vi "main.vi"() -> ()   [LabVIEW 2014]
uses:
  control/DEF-LabVIEW INFO.ctl
  control/DEF-State.ctl
  shared/miscellaneous.llb/miscellaneous.lvlib
panel:
  out "Symbol Found?":bool
  out "Selected Version":string
  out "Version List":string[](array[string])
  out "Symbol Path":path
  out "Symbol Version":string
  out "LabVIEW Info":T1[](array[typedef])
  in  "Cancel":bool
  in  "OK":bool
  in  "LabVIEW List":string(combo)
  in  "file path":path=path "D:/Projects/Personal/Multi-LabVIEW-Selector/Multi-LabVIEW Selector.lvproj" caption="打开文件路径"
  out "CMD line":string caption="命令行参数"
  # "主界面，所有的界面操作都产生消息，推送给Message Framework 处理。"
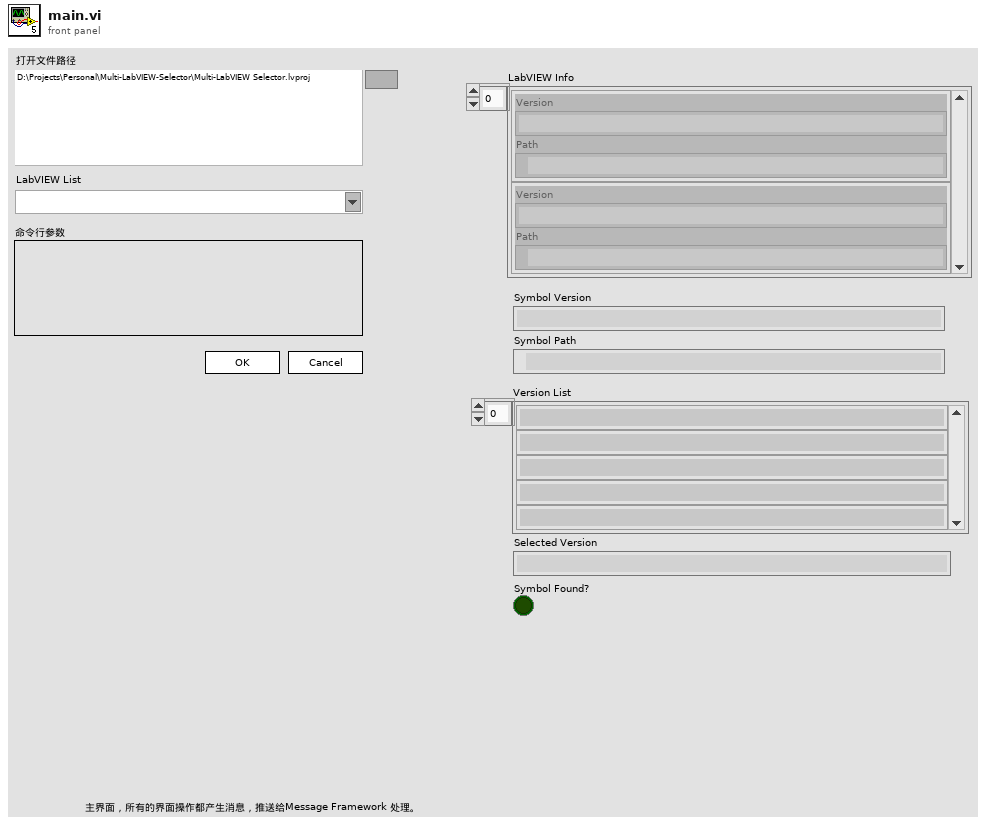
[diagram p1: front panel]
types:
  T1 = typedef "DEF-LabVIEW INFO.ctl" = cluster{"Version":string, "Path":path}
  T2 = typedef "DEF-State.ctl" = enum16{"Get Project Path", "Get Installed LabVIEW Version", "Find New Symbol", "Find Old Symbol", "Replace with New Symbol", "Check If The Symbol Version Exist", "Waiting for User Selection", "Display Information", "Open With Selected LabVIEW Version", "Exit"}
  T3 = cluster{"Project Path":path, "LabVIEW Info":T1[], "Symbol Version":string, "Symbol Path":path, "Version List":string[], "Selected Version":string, "Symbol Found?":bool, "CMD line":string}
  T4 = enum8{"Enabled", "Disabled", "Disabled and Grayed Out"}
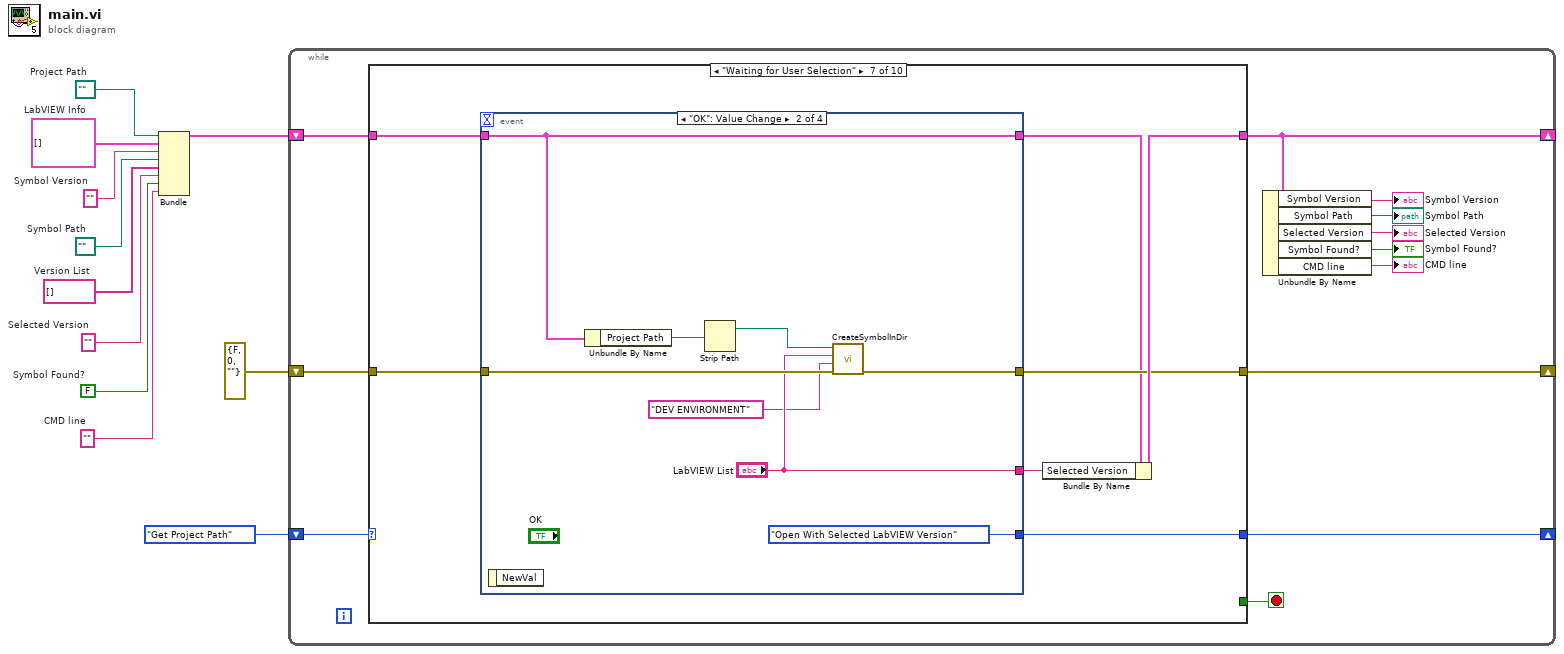
[diagram p0: block diagram]
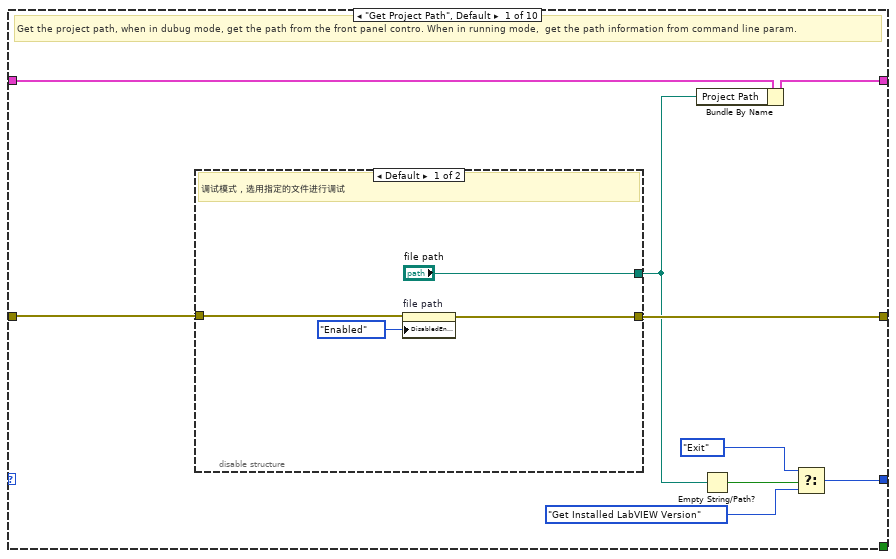
[diagram p2: hidden frame]
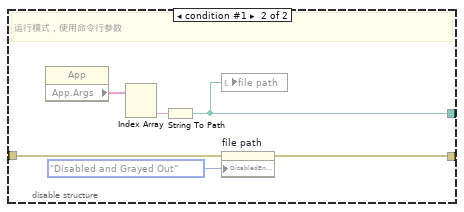
[diagram p3: hidden frame]
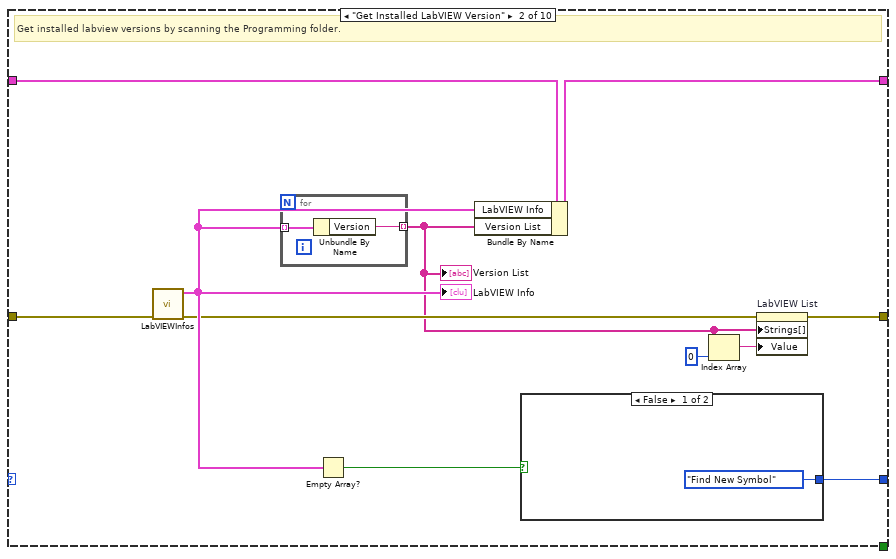
[diagram p4: hidden frame]
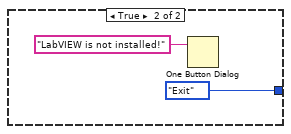
[diagram p5: hidden frame]
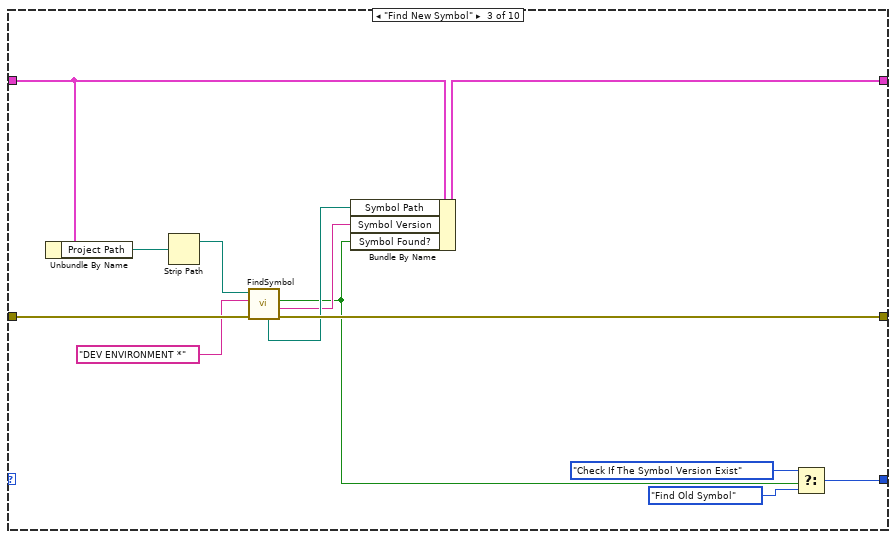
[diagram p6: hidden frame]
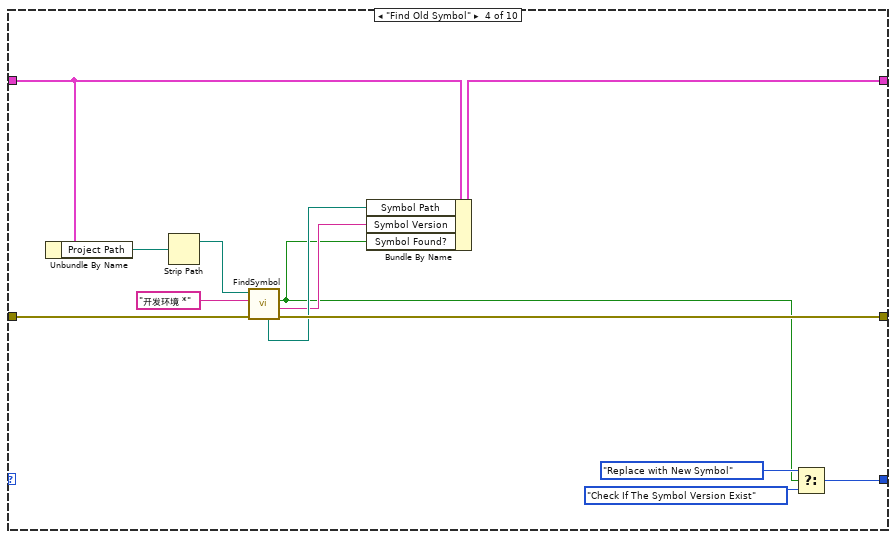
[diagram p7: hidden frame]
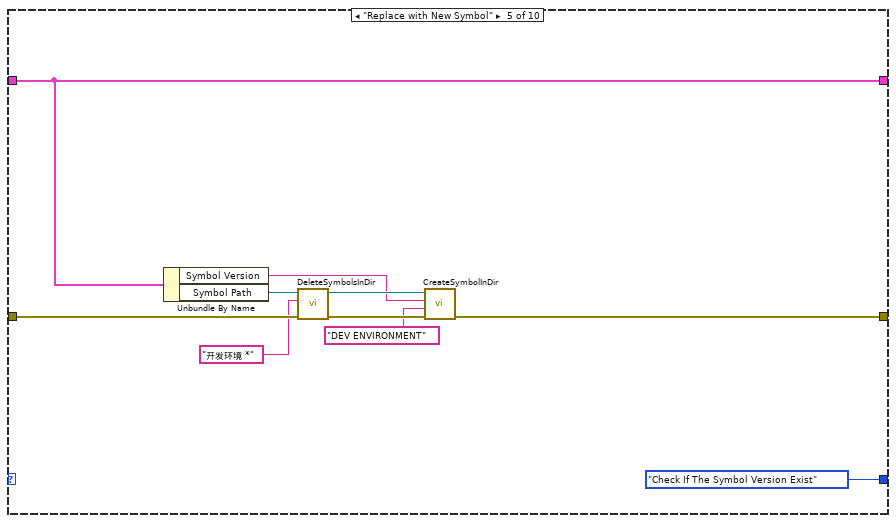
[diagram p8: hidden frame]
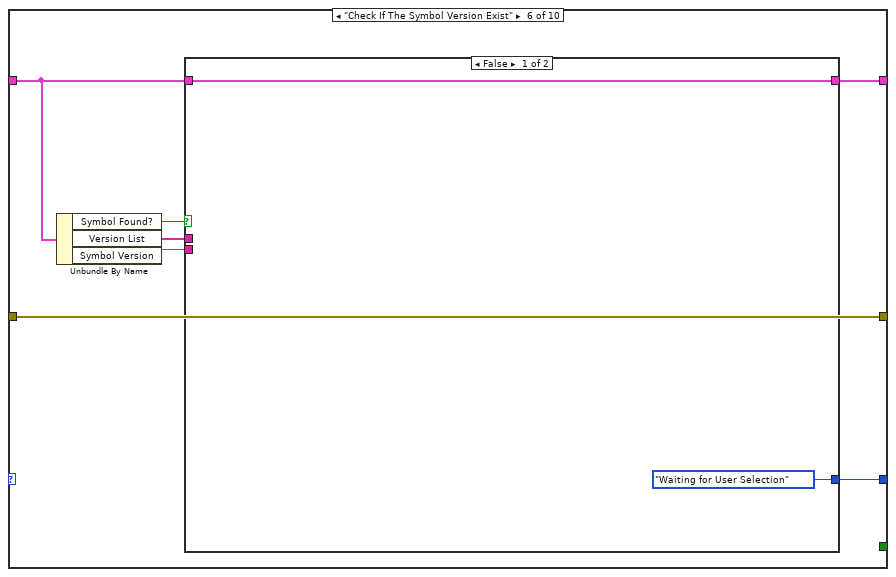
[diagram p9: hidden frame]
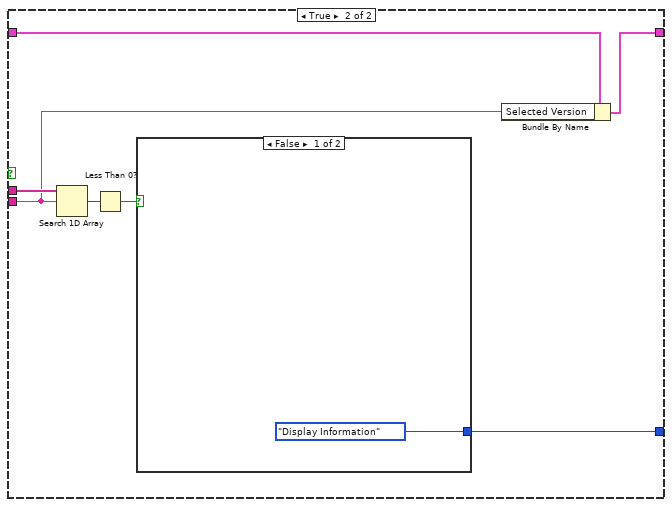
[diagram p10: hidden frame]
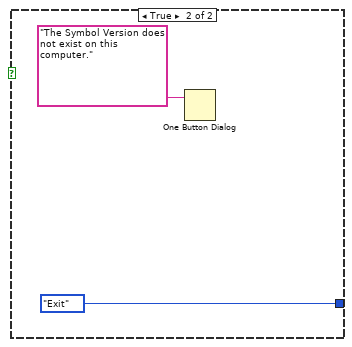
[diagram p11: hidden frame]
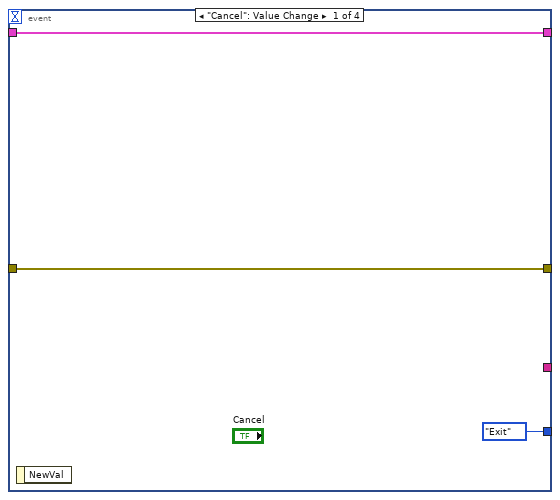
[diagram p12: hidden frame]
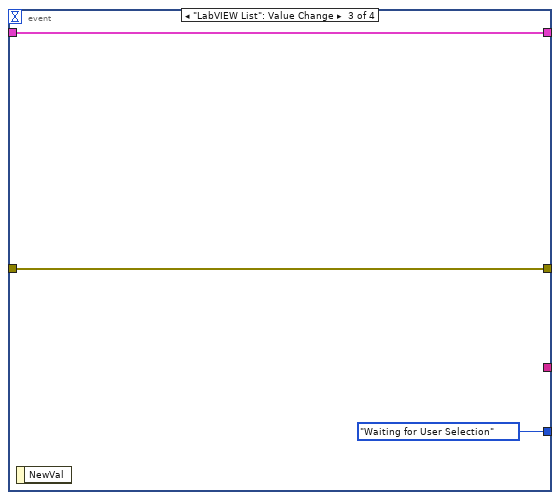
[diagram p13: hidden frame]
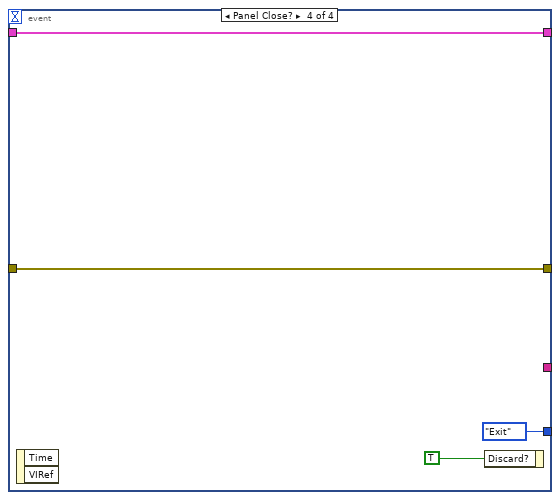
[diagram p14: hidden frame]
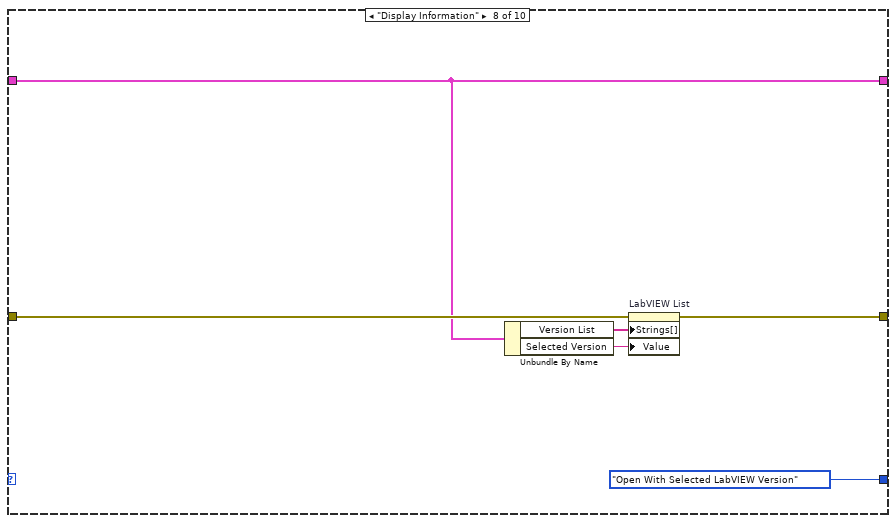
[diagram p15: hidden frame]
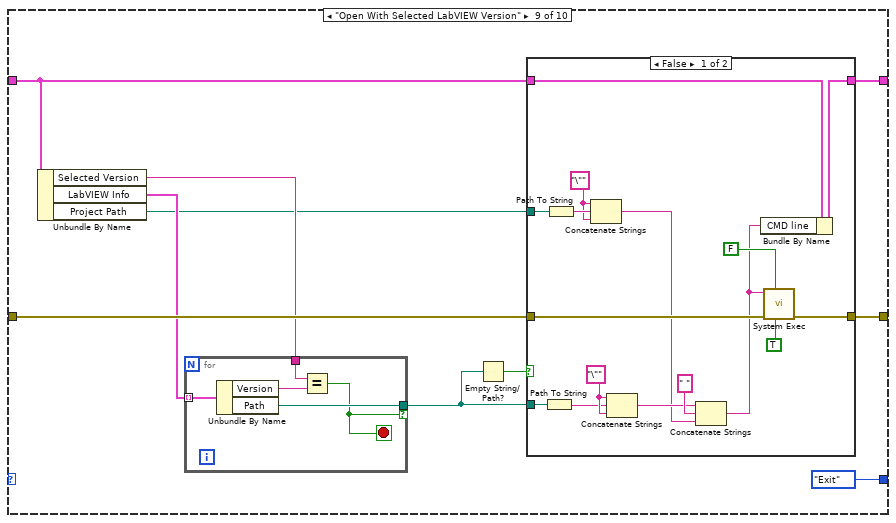
[diagram p16: hidden frame]
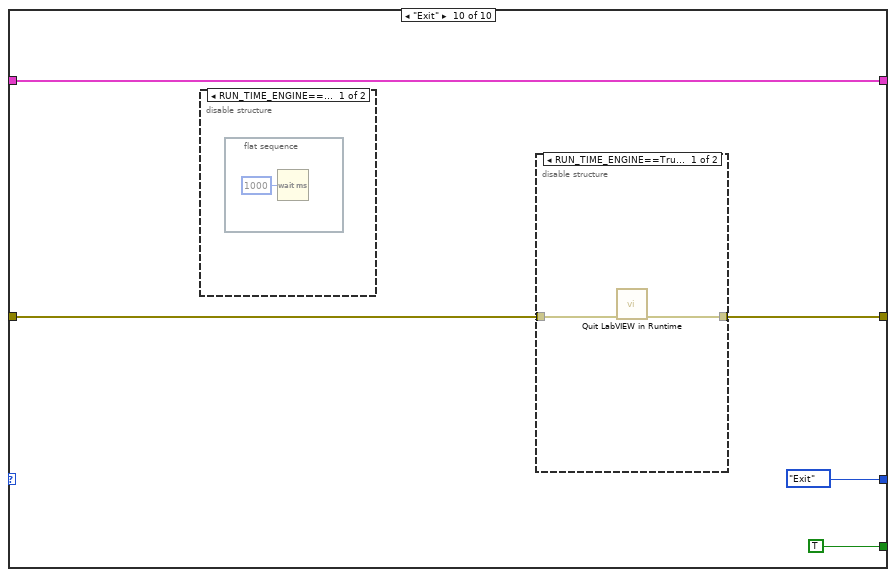
[diagram p18: hidden frame]
diagram:
  w1 = ""  # CMD line
  w2 = FALSE  # Symbol Found?
  w3 = ""  # Selected Version
  w4 = string[] []  # Version List
  w5 = path ""  # Symbol Path
  w6 = ""  # Symbol Version
  w7 = path ""  # Project Path
  w9 = T1[] []  # LabVIEW Info
  n1 = Bundle("Project Path"=w7, "LabVIEW Info"=w9, "Symbol Version"=w6, "Symbol Path"=w5, "Version List"=w4, "Selected Version"=w3, "Symbol Found?"=w2, "CMD line"=w1) -> (w8:T3)  [unwired: 1 in]
  n2 = while {
    shift-right: [w20] -> _
    shift-left: errorcluster {"status"=FALSE, "code"=0, "source"=""} ("error constant") -> [w21]
    shift-right: [w19] -> _
    shift-left: DEF-State."Get Project Path" -> [w23]
    shift-right: [w17] -> _
    shift-left: w8 -> [w18]
    stop <- w22 stop-if-true
    n3 = case shown="\"Waiting for User Selection\"" w23 {
      tunnel: [_ _ _ _ _ _ _ _ _ TRUE] -> w22
      tunnel: w21 -> [w31 w53 w69 w82 w94 w99 w117 w143 w154 w181]
      tunnel: [w32 w44 w65 w77 w89 w99 w116 w144 w153 w180] -> w20
      tunnel: [w29 w49 w66 w78 DEF-State."Check If The Symbol Version Exist" w98 w118 DEF-State."Open With Selected LabVIEW Version" DEF-State."Exit" DEF-State."Exit"] -> w19
      tunnel: w18 -> [w26 w52 w64 w76 w93 w96 w115 w142 w146 w178]
      tunnel: [w25 w51 w62 w74 w93 w95 w120 w142 w145 w178] -> w17
      frame "Get Project Path", Default {
        # "Get the project path, when in dubug mode, get the path from the front panel contro. When in running mode,  get the path information from command line param."
        n4 = disable-structure shown="Default" {
          disable-tunnel: ["file path" w40] -> w24
          disable-tunnel: [w34 w38] -> w32
          disable-tunnel: w31 -> [w33 w37]
          frame condition #0 (active) {
            # "调试模式，选用指定的文件进行调试"
            n5 = property on="file path" class="Path"(error in=w33, "DisabledEnum"=T4."Enabled" ("Disabled")) -> (error out=w34:errorcluster)  [unwired: 1 in, 1 out]
          }
          frame condition #1 {
            # "运行模式，使用命令行参数"
            n6 = property class="App"() -> ("App.Args"=w42:string[])  [unwired: 2 in, 2 out]
            n7 = Index Array(array=w42) -> (element #2=w41:string)  [unwired: 2 in, 1 out]
            n8 = String To Path(string=w41) -> (path=w40:path)
            n9 = local write "file path"(w40) -> ()
            n10 = property on="file path" class="Path"(error in=w37, "DisabledEnum"=T4."Disabled and Grayed Out" ("Disabled")) -> (error out=w38:errorcluster)  [unwired: 1 in, 1 out]
          }
        }
        n11 = Bundle By Name(cluster=w26, "Project Path"=w24) -> (w25:T3)
        n12 = Empty String/Path?(string/path=w24) -> (empty?=w30:bool)
        n13 = Select(t=DEF-State."Exit", s=w30, f=DEF-State."Get Installed LabVIEW Version") -> (s? t:f=w29:T2)
      }
      frame "Get Installed LabVIEW Version" {
        # "Get installed labview versions by scanning the Programming folder."
        n14 = call "LabVIEWInfos.vi"("error in (no error)"=w53) -> ("error out"=w45:errorcluster, "LabVIEW Info"=w48:T1[])  [unwired: 9 in]
        "LabVIEW Info" <- w48
        n15 = for {
          tunnel: w48 -> [w55] mode=indexing
          tunnel: [w54] -> w43 mode=indexing
          n16 = Unbundle By Name(w55) -> ("Version"=w54:string)
        }
        "Version List" <- w43
        n17 = Empty Array?(array=w48) -> (empty?=w50:bool)
        n18 = Bundle By Name(cluster=w52, "LabVIEW Info"=w48, "Version List"=w43) -> (w51:T3)
        n19 = case shown="False" w50 {
          tunnel: [DEF-State."Find New Symbol" DEF-State."Exit"] -> w49
          frame False {
          }
          frame True {
            n20 = One Button Dialog(message="LabVIEW is not installed!") -> ()  [unwired: 1 in, 1 out]
          }
        }
        n21 = Index Array(array=w43, index=0) -> (element=w46:string)
        n22 = property on="LabVIEW List" class="CmbBox"(error in=w45, "Strings[]"=w43, "Value"=w46) -> (error out=w44:errorcluster)  [unwired: 1 in, 1 out]
      }
      frame "Find New Symbol" {
        n23 = Unbundle By Name(w64) -> ("Project Path"=w71:path)
        n24 = Strip Path(path=w71) -> (stripped path=w70:path)  [unwired: 1 out]
        n25 = call "FindSymbol.vi"("error in (no error)"=w69, "pattern"="DEV ENVIRONMENT *" ("prefix"), "path"=w70) -> ("error out"=w65:errorcluster, "Version"=w61:string, "Exits?"=w59:bool, "found path"=w63:path)  [unwired: 4 in, 1 out]
        n26 = Bundle By Name(cluster=w64, "Symbol Path"=w63, "Symbol Version"=w61, "Symbol Found?"=w59) -> (w62:T3)
        n27 = Select(t=DEF-State."Check If The Symbol Version Exist", s=w59, f=DEF-State."Find Old Symbol") -> (s? t:f=w66:T2)
      }
      frame "Find Old Symbol" {
        n28 = Unbundle By Name(w76) -> ("Project Path"=w84:path)
        n29 = Strip Path(path=w84) -> (stripped path=w83:path)  [unwired: 1 out]
        n30 = call "FindSymbol.vi"("error in (no error)"=w82, "pattern"="开发环境 *", "path"=w83) -> ("error out"=w77:errorcluster, "Version"=w73:string, "Exits?"=w72:bool, "found path"=w75:path)  [unwired: 4 in, 1 out]
        n31 = Bundle By Name(cluster=w76, "Symbol Path"=w75, "Symbol Version"=w73, "Symbol Found?"=w72) -> (w74:T3)
        n32 = Select(t=DEF-State."Replace with New Symbol", s=w72, f=DEF-State."Check If The Symbol Version Exist") -> (s? t:f=w78:T2)
      }
      frame "Replace with New Symbol" {
        n33 = Unbundle By Name(w93) -> ("Symbol Version"=w87:string, "Symbol Path"=w92:path)
        n34 = call "DeleteSymbolsInDir.vi"("error in (no error)"=w94, "pattern"="开发环境 *", "dup path"=w92) -> ("error in (no error) (dup)"=w90:errorcluster, "dup path (dup)"=w88:path)  [unwired: 7 in]
        n35 = call "CreateSymbolInDir.vi"("error in"=w90, "prefix"="DEV ENVIRONMENT", "Name"=w87, "Path"=w88) -> ("error out"=w89:errorcluster)  [unwired: 6 in, 1 out]
      }
      frame "Check If The Symbol Version Exist" {
        n36 = Unbundle By Name(w96) -> ("Symbol Found?"=w97:bool, "Version List"=w101:string[], "Symbol Version"=w100:string)
        n37 = case shown="False" w97 {
          tunnel: w101 -> [_ w109]
          tunnel: w100 -> [_ w104]
          tunnel: [DEF-State."Waiting for User Selection" w108] -> w98
          tunnel: w96 -> [w102 w106]
          tunnel: [w102 w105] -> w95
          frame False {
          }
          frame True {
            n38 = Search 1D Array(1D array=w109, element=w104) -> (index of element=w110:i32)  [unwired: 1 in]
            n39 = Less Than 0?(x=w110) -> (x < 0?=w107:bool)
            n40 = case shown="False" w107 {
              tunnel: [DEF-State."Display Information" DEF-State."Exit"] -> w108
              frame False {
              }
              frame True {
                n41 = One Button Dialog(message="The Symbol Version does not exist on this computer.") -> ()  [unwired: 1 in, 1 out]
              }
            }
            n42 = Bundle By Name(cluster=w106, "Selected Version"=w104) -> (w105:T3)
          }
        }
      }
      frame "Waiting for User Selection" {
        n43 = event shown="[1] \"OK\": Value Change" {
          selector: _ -> [_ _ _ _]
          dyn-events: _ -> [_ _ _ _]
          timeout: _ -> [_ _ _ _]
          tunnel: [_ "LabVIEW List" _ _] -> w119
          tunnel: [DEF-State."Exit" DEF-State."Open With Selected LabVIEW Version" DEF-State."Waiting for User Selection" DEF-State."Exit"] -> w118
          tunnel: w117 -> [w122 w130 w133 w136]
          tunnel: [w122 w129 w133 w136] -> w116
          tunnel: w115 -> [w121 w128 w132 w135]
          tunnel: [w121 w128 w132 w135] -> w114
          event "Cancel": Value Change {
            n44 = event-data() -> ()  [unwired: 1 in, 1 out]
          }
          event "OK": Value Change {
            n45 = event-data() -> ()  [unwired: 1 in, 1 out]
            n46 = Unbundle By Name(w128) -> ("Project Path"=w127:path)
            n47 = Strip Path(path=w127) -> (stripped path=w126:path)  [unwired: 1 out]
            n48 = call "CreateSymbolInDir.vi"("error in"=w130, "prefix"="DEV ENVIRONMENT", "Name"="LabVIEW List", "Path"=w126) -> ("error out"=w129:errorcluster)  [unwired: 6 in, 1 out]
          }
          event "LabVIEW List": Value Change {
            n49 = event-data() -> ()  [unwired: 1 in, 1 out]
          }
          event Panel Close? {
            n50 = event-data() -> ()  [unwired: 1 in, 2 out]
            n51 = event-data("Discard?"=TRUE) -> ()  [unwired: 1 in, 1 out]
          }
        }
        n52 = Bundle By Name(cluster=w114, "Selected Version"=w119) -> (w120:T3)
      }
      frame "Display Information" {
        n53 = Unbundle By Name(w142) -> ("Version List"=w141:string[], "Selected Version"=w140:string)
        n54 = property on="LabVIEW List" class="CmbBox"(error in=w143, "Strings[]"=w141, "Value"=w140) -> (error out=w144:errorcluster)  [unwired: 1 in, 1 out]
      }
      frame "Open With Selected LabVIEW Version" {
        n55 = Unbundle By Name(w146) -> ("Selected Version"=w150:string, "LabVIEW Info"=w149:T1[], "Project Path"=w147:path)
        n56 = for {
          tunnel: w149 -> [w177] mode=indexing
          tunnel: [w175] -> w152 if=w173
          tunnel: w150 -> [w174]
          stop <- w173 stop-if-true
          n57 = Unbundle By Name(w177) -> ("Version"=w176:string, "Path"=w175:path)
          n58 = Equal?(x=w174, y=w176) -> (x = y?=w173:bool)
        }
        n59 = Empty String/Path?(string/path=w152) -> (empty?=w151:bool)
        n60 = case shown="False" w151 {
          tunnel: w154 -> [w170 w172]
          tunnel: w152 -> [w169 _]
          tunnel: [w159 w172] -> w153
          tunnel: w147 -> [w158 _]
          tunnel: w146 -> [w157 w171]
          tunnel: [w156 w171] -> w145
          frame False {
            w166 = "\"" ("string")
            w167 = "\"" ("string")
            n61 = Path To String(path=w169) -> (string=w165:string)
            n62 = Path To String(path=w158) -> (string=w168:string)
            n63 = Concatenate Strings(w167, w168, w167) -> (w162:string)
            n64 = Concatenate Strings(w166, w165, w166) -> (w163:string)
            n65 = Concatenate Strings(w163, " " ("string"), w162) -> (w155:string)
            n66 = Bundle By Name(cluster=w157, "CMD line"=w155) -> (w156:T3)
            n67 = call <vilib>:"System Exec.vi"("run minimized? (F)"=TRUE, "wait until completion? (T)"=FALSE, "error in (no error)"=w170, "command line"=w155) -> ("error out"=w159:errorcluster)  [unwired: 4 in, 3 out]
          }
          frame True {
          }
        }
      }
      frame "Exit" {
        n68 = disable-structure shown="RUN_TIME_ENGINE==True" {
          frame condition #0 {
            n69 = flat-sequence {
              frame #0 {
                n70 = Wait (ms)(milliseconds to wait=u32 1000) -> ()  [unwired: 1 out]
              }
            }
          }
          frame condition #1 (active) {
          }
        }
        n71 = disable-structure shown="RUN_TIME_ENGINE==True" {
          disable-tunnel: w181 -> [w184 w186]
          disable-tunnel: [w185 w186] -> w180
          frame condition #0 {
            n72 = call "Quit LabVIEW in Runtime.vi"("error in (no error)"=w184) -> ("error in (no error) (dup)"=w185:errorcluster)  [unwired: 10 in]
          }
          frame condition #1 (active) {
          }
        }
      }
    }
    n73 = Unbundle By Name(w17) -> ("Symbol Version"=→"Symbol Version":string, "Symbol Path"=→"Symbol Path":path, "Selected Version"=→"Selected Version":string, "Symbol Found?"=→"Symbol Found?":bool, "CMD line"=→"CMD line":string)
  }
